vi "Write Blink.vi"(8 "error in (no error)":errorcluster, 10 "Blink? Ref":bool, 11 "Power Meter Display in":refnum<class "Power Meter Display.lvclass">) -> (0 "error out":errorcluster, 3 "Power Meter Display out":refnum<class "Power Meter Display.lvclass">)   [LabVIEW 2012, in "Display Panel.lvlib" / "Power Meter Display.lvclass"]
uses:
  Power Meter Display.lvclass
  Power Meter Display.lvclass/Power Meter Display.ctl
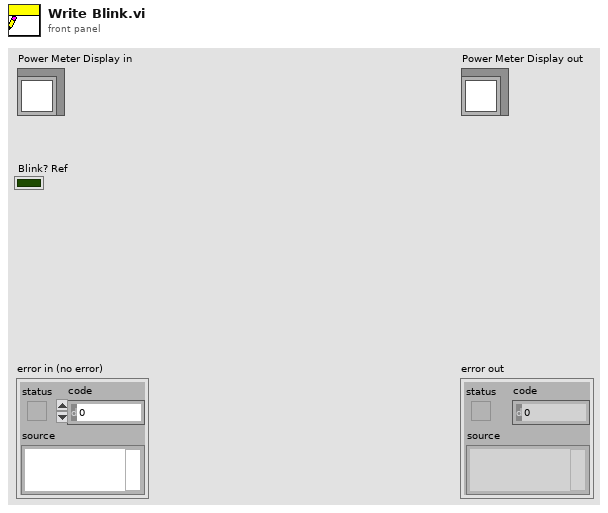
[diagram p1: front panel]
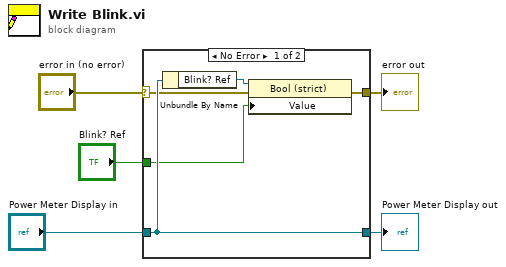
[diagram p0: block diagram]
diagram:
  n1 = case shown="No Error" "error in (no error)" {
    selector: "error in (no error)" -> [w8 w11]
    tunnel: [w7 w11] -> w4
    tunnel: [w10 w12] -> w2
    tunnel: "Power Meter Display in" -> [w10 w12]
    tunnel: "Blink? Ref" -> [w6 _]
    frame No Error {
      n2 = Unbundle By Name(w10) -> ("Blink? Ref"=w9:refnum<vi>)
      n3 = property class="Bool (strict)"(reference=w9, error in=w8, "Value"=w6) -> (error out=w7:errorcluster)  [unwired: 1 out]
    }
    frame Error {
    }
  }
  "error out" <- w4
  "Power Meter Display out" <- w2
